vi "do_peaks_match_subvi.vi"(0 "derivative in":waveform(dbl), 1 "X in":waveform(dbl), 4 "sampling info":cluster{"Fs":dbl, "#s":dbl}) -> (7 "X out":waveform(dbl), 8 "peaks match":bool)   [LabVIEW 2015]
uses:
  <vilib>/Analysis/3filter.llb/Butterworth Filter (DBL).vi
  <vilib>/Analysis/NI_AALBase.lvlib
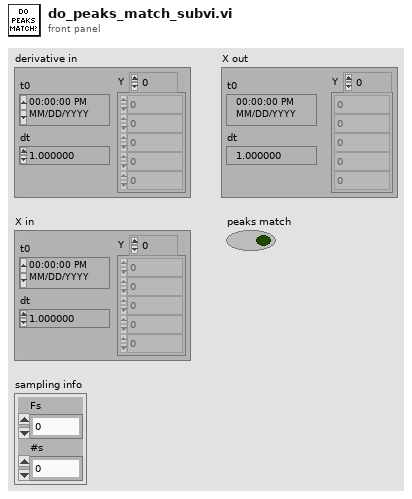
[diagram p1: front panel]
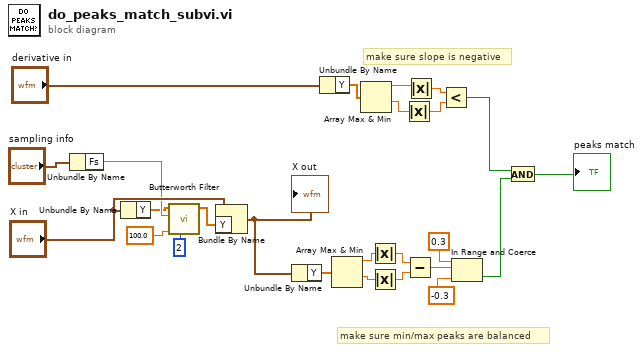
[diagram p0: block diagram]
diagram:
  # "make sure min/max peaks are balanced"
  # "make sure slope is negative"
  n1 = Unbundle By Name("sampling info") -> ("Fs"=w22:dbl)
  n2 = Unbundle By Name("X in") -> ("Y"=w18:dbl[])
  n3 = call-poly <vilib>:"Butterworth Filter.vi"("order"=2, "low cutoff freq: fl"=100.0, "sampling freq: fs"=w22, "X"=w18) -> ("Filtered X"=w19:dbl[])  [unwired: 4 in, 1 out]
  n4 = Bundle By Name(cluster="X in", "Y"=w19) -> (w24:waveform(dbl))
  "X out" <- w24
  n5 = Unbundle By Name(w24) -> ("Y"=w2:dbl[])
  n6 = Unbundle By Name("derivative in") -> ("Y"=w10:dbl[])
  n7 = Array Max & Min(array=w2) -> (max value=w4:dbl, min value=w3:dbl)  [unwired: 2 out]
  n8 = Array Max & Min(array=w10) -> (max value=w11:dbl, min value=w12:dbl)  [unwired: 2 out]
  n9 = Absolute Value(x=w4) -> (abs(x)=w5:dbl)
  n10 = Absolute Value(x=w3) -> (abs(x)=w6:dbl)
  n11 = Absolute Value(x=w12) -> (abs(x)=w14:dbl)
  n12 = Subtract(x=w5, y=w6) -> (x-y=w15:dbl)
  n13 = Absolute Value(x=w11) -> (abs(x)=w13:dbl)
  n14 = Less?(x=w13, y=w14) -> (x < y?=w16:bool)
  n15 = In Range and Coerce(upper limit=0.3, x=w15, lower limit=-0.3) -> (In Range?=w17:bool)  [unwired: 1 out]
  n16 = And(x=w16, y=w17) -> (x .and. y?=→"peaks match":bool)
